vi "NumPesoCalRequest.vi"() -> (0 "NumProm":dbl=100.0 format="%.2f")   [LabVIEW 2013]
panel:
  in  "Peso de calibración (mg)":dbl=100.0 min=0.0 max=100.0 step=0.001 format="%.3f"
  in  "OK Button":bool
  # "Introduzca nuevo peso de calibración (mg)"
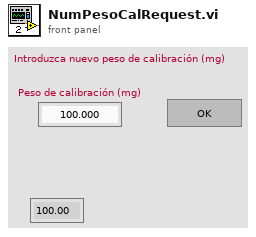
[diagram p1: front panel]
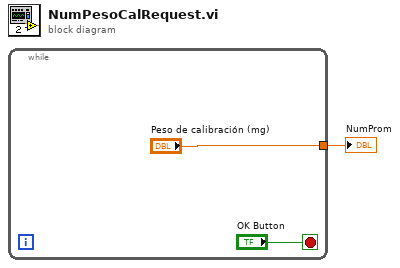
[diagram p0: block diagram]
diagram:
  n1 = while {
    tunnel: ["Peso de calibración (mg)"] -> w1
    stop <- "OK Button" stop-if-true
  }
  "NumProm" <- w1
